vi "searchInXmlNodes2.vi"(8 "error in (no error)":errorcluster, 9 "searchElementName":string, 10 "searchElementIn":string, 11 "xmlNode in":refnum<class "xmlNode.lvclass">) -> (0 "error out":errorcluster, 2 "arrayXmlNodes":refnum<class "xmlNode.lvclass">[](array[class]), 3 "xmlNode out":refnum<class "xmlNode.lvclass">)   [LabVIEW 2011, in "Tools.lvlib" / "xml.lvlib" / "xmlNode.lvclass"]
uses:
  xmlNode.lvclass
  XmlParser.lvclass
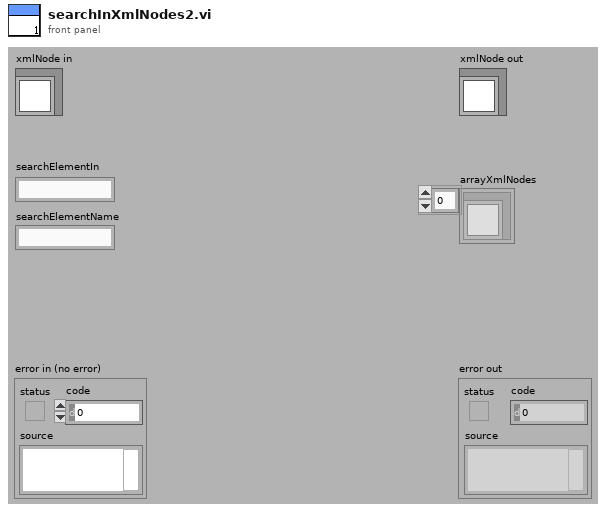
[diagram p1: front panel]
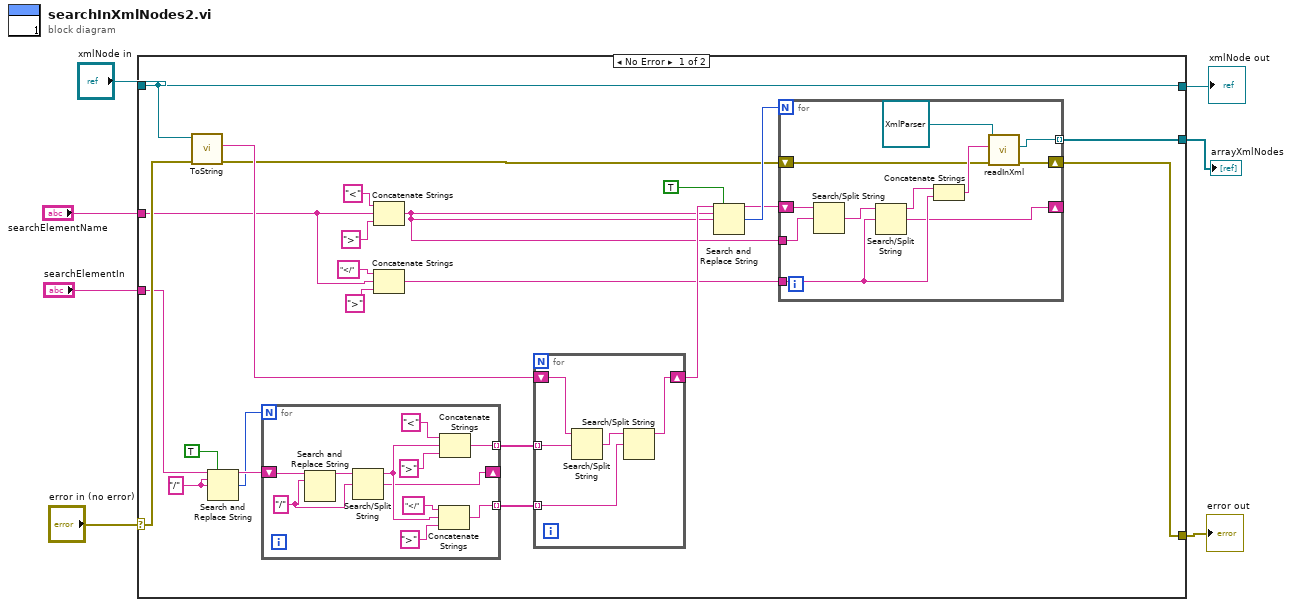
[diagram p0: block diagram]
diagram:
  n1 = case shown="No Error" "error in (no error)" {
    selector: "error in (no error)" -> [w27 w60]
    tunnel: [w11 w60] -> w1
    tunnel: [w28 w59] -> w5
    tunnel: "xmlNode in" -> [w28 w59]
    tunnel: "searchElementIn" -> [w10 _]
    tunnel: "searchElementName" -> [w18 _]
    tunnel: [w12 _] -> w2
    frame No Error {
      w29 = "/"
      n2 = call-dynamic "ToString.vi"("error in (no error)"=w27, "xmlNode in"=w28) -> ("error out"=w13:errorcluster, "xml"=w26:string)  [unwired: 7 in, 1 out]
      n3 = Search and Replace String(replace all?=TRUE, input string=w10, search string=w29, replace string=w29) -> (result string=w31:string, number of replacements=w30:i32)  [unwired: 4 in, 2 out]
      n4 = for {
        N: w30 -> [_]
        tunnel: [w50] -> w25 mode=indexing
        tunnel: [w49] -> w24 mode=indexing
        shift-right: [w48] -> _
        shift-left: w31 -> [w58]
        w57 = "/"
        n5 = Search and Replace String(input string=w58, search string=w57) -> (result string=w56:string)  [unwired: 6 in, 3 out]
        n6 = Search/Split String(string=w56, search string/char (-)=w57) -> (substring before match=w51:string, match + rest of string=w48:string)  [unwired: 1 in, 1 out]
        n7 = Concatenate Strings("</", w51, ">") -> (w49:string)
        n8 = Concatenate Strings("<", w51, ">") -> (w50:string)
      }
      n9 = Concatenate Strings("<", w18, ">") -> (w15:string)
      n10 = Concatenate Strings("</", w18, ">") -> (w14:string)
      n11 = for {
        tunnel: w25 -> [w46] mode=indexing
        tunnel: w24 -> [w44] mode=indexing
        shift-right: [w43] -> w23
        shift-left: w26 -> [w47]
        n12 = Search/Split String(string=w47, search string/char (-)=w46) -> (match + rest of string=w45:string)  [unwired: 1 in, 2 out]
        n13 = Search/Split String(string=w45, search string/char (-)=w44) -> (substring before match=w43:string)  [unwired: 1 in, 2 out]
      }
      n14 = Search and Replace String(replace all?=TRUE, input string=w23, search string=w15, replace string=w15) -> (result string=w16:string, number of replacements=w17:i32)  [unwired: 4 in, 2 out]
      n15 = for {
        N: w17 -> [_]
        tunnel: w15 -> [w41]
        tunnel: w14 -> [w39]
        shift-right: [w34] -> _
        shift-left: w16 -> [w42]
        tunnel: [w32] -> w12 mode=indexing
        shift-right: [w33] -> w11
        shift-left: w13 -> [w36]
        n16 = Search/Split String(string=w42, search string/char (-)=w41) -> (match + rest of string=w40:string)  [unwired: 1 in, 2 out]
        n17 = Search/Split String(string=w40, search string/char (-)=w39) -> (substring before match=w35:string, match + rest of string=w34:string)  [unwired: 1 in, 1 out]
        n18 = Concatenate Strings(w35, w39) -> (w37:string)
        n19 = call "readInXml.vi"("error in (no error)"=w36, "xmlString"=w37, "XmlParser in"=refnum<class "XmlParser.lvclass"> refnum ("Tools.lvlib:XmlParser.lvclass")) -> ("error out"=w33:errorcluster, "xmlNode"=w32:refnum<class "xmlNode.lvclass">)  [unwired: 6 in, 1 out]
      }
    }
    frame Error {
    }
  }
  "error out" <- w1
  "xmlNode out" <- w5
  "arrayXmlNodes" <- w2
